vi "Get AI Signal - Multiple.vi"(0 "reference in":refnum<class "AI.lvclass">, 3 "AI Channel Numbers (Zero Based)":i32[](array[numeric]), 4 "Zero Threshold":dbl, 5 "error in (no error)":errorcluster) -> (11 "AI Channel Signal is Zero":bool[](array[boolean]), 14 "reference out":refnum<class "AI.lvclass">, 16 "AI Channel Readings":dbl[][](array[numeric]), 17 "AI Channel Average":dbl[](array[numeric]), 18 "AI Channel Standard Deviation":dbl[](array[numeric]), 19 "error out":errorcluster)   [LabVIEW 2017, in "AI.lvclass"]
uses:
  AI.lvclass
  <vilib>/Analysis/NI_AALBase.lvlib
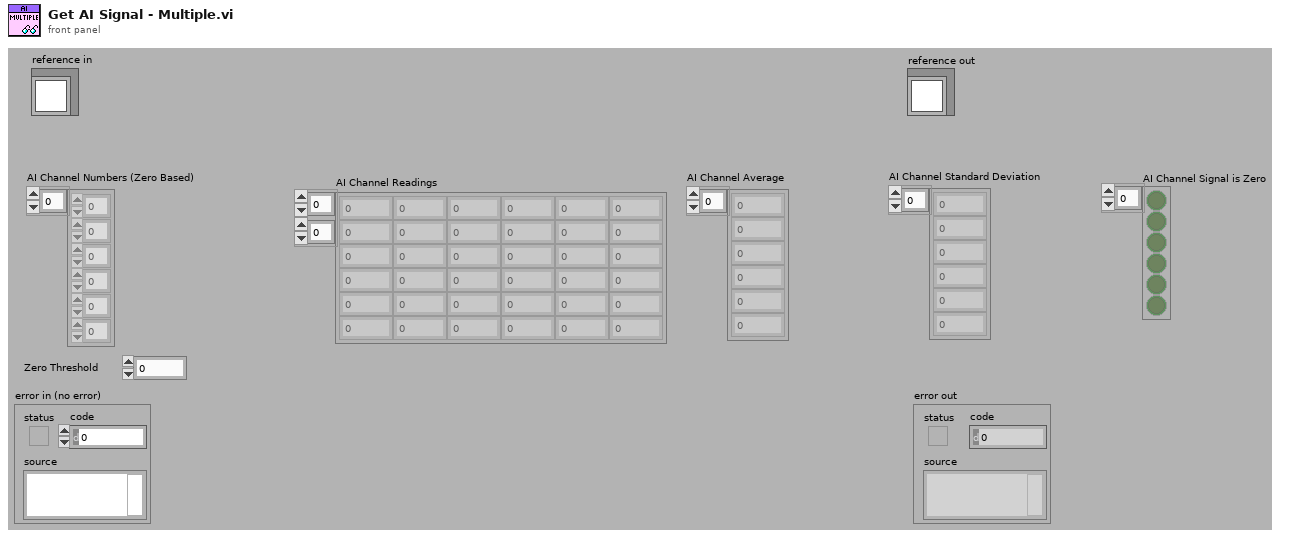
[diagram p1: front panel]
types:
  T1 = typedef "AI.lvclass/ObjectAttributes.ctl" = cluster{"AI Task":refnum<k21>, "AI On/Off Status":bool, "AI Sampling Rate (Samples/Seconds)":u32, "Number of AI Samples Per Channel":i32, "AI Voltage Range":u8, "AI Readings":dbl[][], "Number of AI Modules":i32, "Number of Total AI Channels":i32, "AI Module Names (NI-Max Name)":string[], "Number of Channels Per AI  Module":i32[], "AI VI Reference":refnum<vi>}
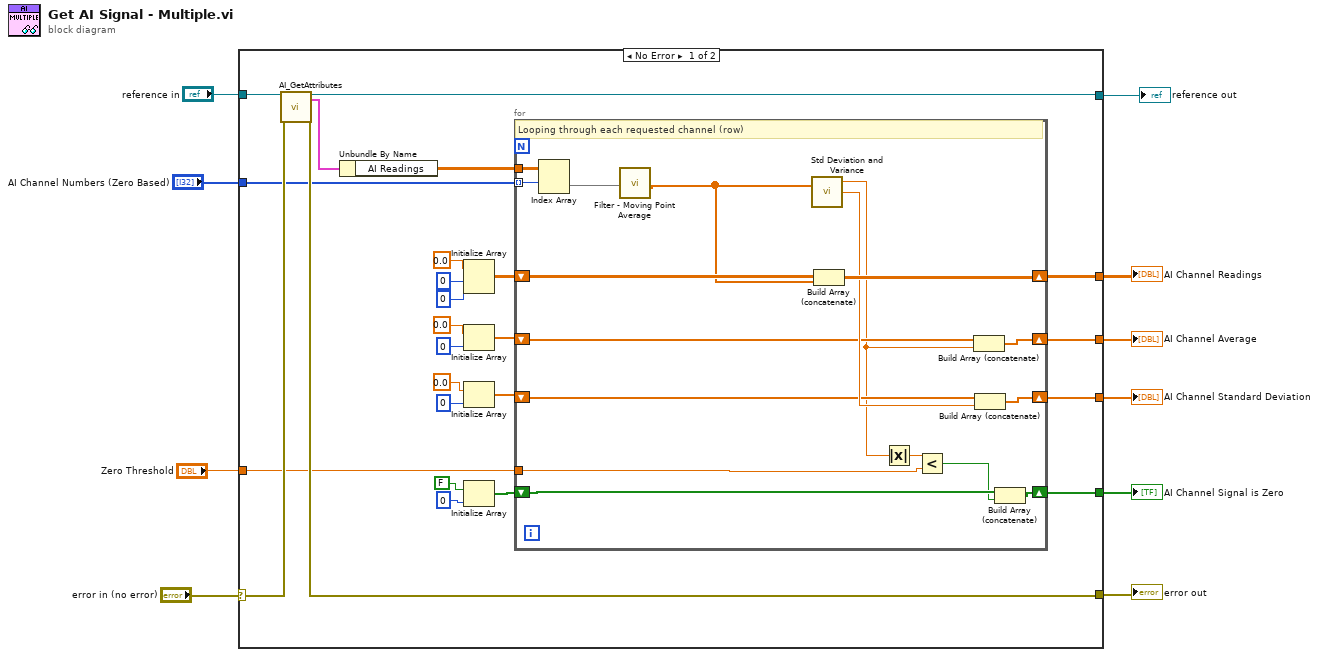
[diagram p0: block diagram]
diagram:
  n1 = case shown="No Error" "error in (no error)" {
    selector: "error in (no error)" -> [w34 w54]
    tunnel: [w32 w54] -> w9
    tunnel: [w33 w53] -> w7
    tunnel: "reference in" -> [w35 w53]
    tunnel: "AI Channel Numbers (Zero Based)" -> [w31 _]
    tunnel: [w30 _] -> w5
    tunnel: [w29 _] -> w4
    tunnel: [w28 _] -> w3
    tunnel: [w27 _] -> w2
    tunnel: "Zero Threshold" -> [w11 _]
    frame No Error {
      n2 = call "AI_GetAttributes.vi"("reference in"=w35, "error in (no error)"=w34) -> ("reference out"=w33:refnum<class "AI.lvclass">, "Data"=w12:T1, "error out"=w32:errorcluster)  [unwired: 14 in, 1 out]
      n3 = Unbundle By Name(w12) -> ("AI Readings"=w26:dbl[][])
      n4 = Initialize Array(0.0 ("element"), 0 ("dimension size"), 0 ("dimension size")) -> (w23:dbl[][])
      n5 = Initialize Array(0.0 ("element"), 0 ("dimension size")) -> (w19:dbl[])
      n6 = Initialize Array(0.0 ("element"), 0 ("dimension size")) -> (w16:dbl[])
      n7 = Initialize Array(FALSE, 0 ("dimension size")) -> (w14:bool[])
      n8 = for {
        tunnel: w26 -> [w52]
        tunnel: w31 -> [w51] mode=indexing
        shift-right: [w49] -> w30
        shift-left: w23 -> [w50]
        shift-right: [w46] -> w29
        shift-left: w19 -> [w47]
        shift-right: [w44] -> w28
        shift-left: w16 -> [w45]
        shift-right: [w42] -> w27
        shift-left: w14 -> [w43]
        tunnel: w11 -> [w38]
        # "Looping through each requested channel (row)"
        n9 = Index Array(array=w52, index (row)=w51) -> (element=w37:dbl[])  [unwired: 1 in]
        n10 = call "Filter - Moving Point Average.vi"("Analog Signal"=w37) -> ("Filtered Analog Signal"=w36:dbl[])  [unwired: 10 in]
        n11 = call <vilib>:"Std Deviation and Variance.vi"("X"=w36) -> ("mean"=w41:dbl, "standard deviation"=w48:dbl)  [unwired: 1 in, 1 out]
        n12 = Build Array (concatenate)(w50, w36) -> (w49:dbl[][])
        n13 = Absolute Value(x=w41) -> (abs(x)=w40:dbl)
        n14 = Less?(x=w40, y=w38) -> (x < y?=w39:bool)
        n15 = Build Array (concatenate)(w47, w41) -> (w46:dbl[])
        n16 = Build Array (concatenate)(w45, w48) -> (w44:dbl[])
        n17 = Build Array (concatenate)(w43, w39) -> (w42:bool[])
      }
    }
    frame Error {
    }
  }
  "error out" <- w9
  "reference out" <- w7
  "AI Channel Readings" <- w5
  "AI Channel Standard Deviation" <- w3
  "AI Channel Average" <- w4
  "AI Channel Signal is Zero" <- w2
